vi "Read._Overload.vi"(0 "Index":i32, 1 "Choose_Device":T1(ring), 2 "error in (no error)":errorcluster) -> (3 "Index_Out":i32, 4 "Overload":bool, 5 "Device_type":T1(ring), 6 "error out":errorcluster)   [LabVIEW 2010, in "FEMTO_LUCI-10.lvlib"]
doc: "This function reads the overload of the selected device."
uses:
  <userlib>/FEMTO/FEMTO_LUCI-10.lvlib
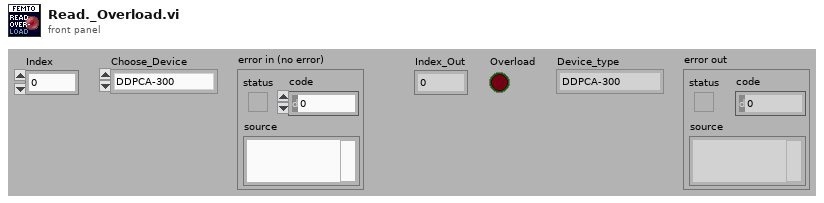
[diagram p1: front panel]
types:
  T1 = enum16{"DDPCA-300", "DLPCA-200", "DHPCA-100", "OE-200", "LIA-MV-150-S", "LIA-MV-150-D", "LIA-MV-200-L", "LIA-MV-200-H", "LIA-MVD-200-L", "LIA-MVD-200-H", "DLPVA-100-BUN-S", "DLPVA-100-BLN-S", "DLPVA-100-B-S", "DLPVA-100-B-D", "DLPVA-100-F-S", "DLPVA-100-F-D", "DHPVA-100", "DHPVA-200", "DUPVA-1-60", "DUPVA-1-70"}
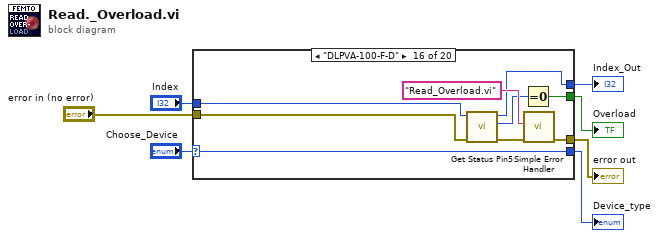
[diagram p0: block diagram]
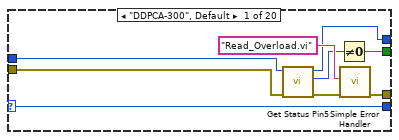
[diagram p2: hidden frame]
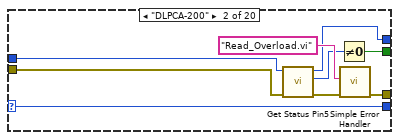
[diagram p3: hidden frame]
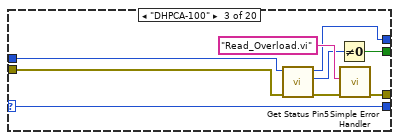
[diagram p4: hidden frame]
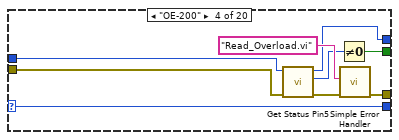
[diagram p5: hidden frame]
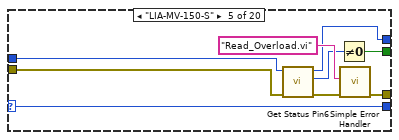
[diagram p6: hidden frame]
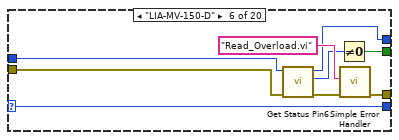
[diagram p7: hidden frame]
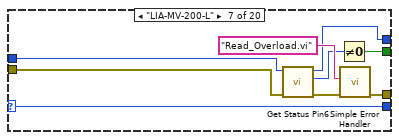
[diagram p8: hidden frame]
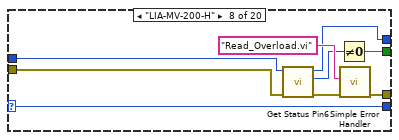
[diagram p9: hidden frame]
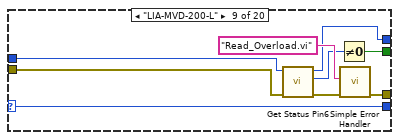
[diagram p10: hidden frame]
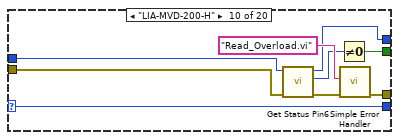
[diagram p11: hidden frame]
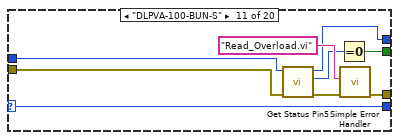
[diagram p12: hidden frame]
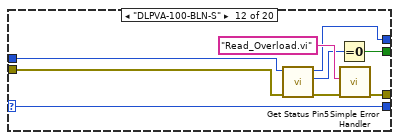
[diagram p13: hidden frame]
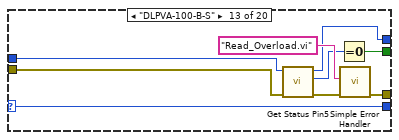
[diagram p14: hidden frame]
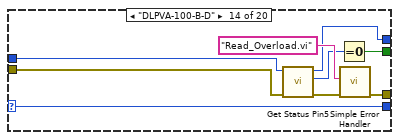
[diagram p15: hidden frame]
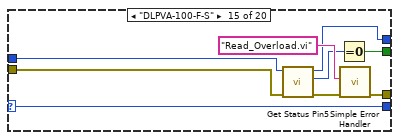
[diagram p16: hidden frame]
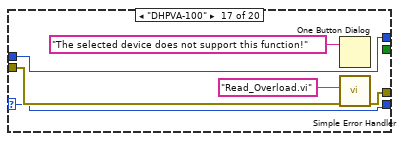
[diagram p17: hidden frame]
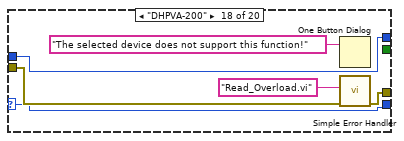
[diagram p18: hidden frame]
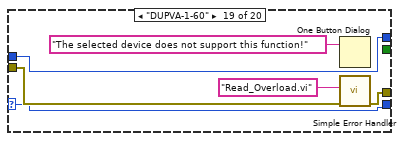
[diagram p19: hidden frame]
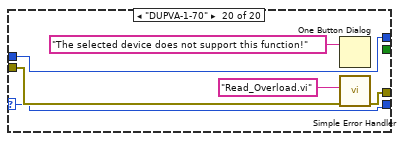
[diagram p20: hidden frame]
diagram:
  n1 = case shown="\"DLPVA-100-F-D\"" "Choose_Device" {
    selector: "Choose_Device" -> [w14 w24 w32 w41 w50 w59 w68 w77 w86 w95 w104 w113 w122 w131 w141 w149 w154 w160 w166 w172]
    tunnel: "error in (no error)" -> [w13 w18 w27 w36 w45 w54 w63 w74 w85 w93 w99 w111 w120 w126 w136 w144 w156 w162 w168 w174]
    tunnel: [w15 w25 w34 w42 w51 w60 w69 w78 w87 w96 w105 w114 w123 w132 w134 w150 w155 w161 w167 w173] -> w3
    tunnel: [w14 w24 w32 w41 w50 w59 w68 w77 w86 w95 w104 w113 w122 w131 w141 w149 w154 w160 w166 w172] -> w4
    tunnel: "Index" -> [w11 w21 w30 w39 w47 w56 w65 w72 w83 w91 w102 w107 w118 w129 w139 w147 w153 w159 w165 w171]
    tunnel: [w10 w20 w29 w38 w46 w55 w64 w71 w82 w90 w101 w108 w117 w128 w138 w146 w153 w159 w165 w171] -> w6
    tunnel: [w8 w19 w28 w37 w48 w57 w66 w75 w80 w89 w100 w109 w116 w127 w137 w145 _ _ _ _] -> w7
    frame "DDPCA-300", Default {
      n2 = call <userlib>:"Get Status Pin5.vi"("error in (no error)"=w13, "index"=w11) -> ("error out"=w12:errorcluster, "status out"=w9:i32, "index_out"=w10:i32)  [unwired: 7 out]
      n3 = Not Equal To 0?(x=w9) -> (x != 0?=w8:bool)
      n4 = call <vilib>:"Simple Error Handler.vi"("error source (\" \")"="Read_Overload.vi" ("error source (\" \")"), "error in (no error)"=w12) -> ("error out"=w15:errorcluster)  [unwired: 1 in, 6 out]
    }
    frame "DLPCA-200" {
      n5 = call <userlib>:"Get Status Pin5.vi"("error in (no error)"=w18, "index"=w21) -> ("error out"=w17:errorcluster, "status out"=w22:i32, "index_out"=w20:i32)  [unwired: 7 out]
      n6 = Not Equal To 0?(x=w22) -> (x != 0?=w19:bool)
      n7 = call <vilib>:"Simple Error Handler.vi"("error source (\" \")"="Read_Overload.vi" ("error source (\" \")"), "error in (no error)"=w17) -> ("error out"=w25:errorcluster)  [unwired: 1 in, 6 out]
    }
    frame "DHPCA-100" {
      n8 = call <userlib>:"Get Status Pin5.vi"("error in (no error)"=w27, "index"=w30) -> ("error out"=w26:errorcluster, "status out"=w31:i32, "index_out"=w29:i32)  [unwired: 7 out]
      n9 = Not Equal To 0?(x=w31) -> (x != 0?=w28:bool)
      n10 = call <vilib>:"Simple Error Handler.vi"("error source (\" \")"="Read_Overload.vi" ("error source (\" \")"), "error in (no error)"=w26) -> ("error out"=w34:errorcluster)  [unwired: 1 in, 6 out]
    }
    frame "OE-200" {
      n11 = call <userlib>:"Get Status Pin5.vi"("error in (no error)"=w36, "index"=w39) -> ("error out"=w35:errorcluster, "status out"=w40:i32, "index_out"=w38:i32)  [unwired: 7 out]
      n12 = Not Equal To 0?(x=w40) -> (x != 0?=w37:bool)
      n13 = call <vilib>:"Simple Error Handler.vi"("error source (\" \")"="Read_Overload.vi" ("error source (\" \")"), "error in (no error)"=w35) -> ("error out"=w42:errorcluster)  [unwired: 1 in, 6 out]
    }
    frame "LIA-MV-150-S" {
      n14 = call <userlib>:"Get Status Pin6.vi"("error in (no error)"=w45, "index"=w47) -> ("error out"=w44:errorcluster, "status out"=w49:i32, "index_out"=w46:i32)  [unwired: 7 out]
      n15 = Not Equal To 0?(x=w49) -> (x != 0?=w48:bool)
      n16 = call <vilib>:"Simple Error Handler.vi"("error source (\" \")"="Read_Overload.vi" ("error source (\" \")"), "error in (no error)"=w44) -> ("error out"=w51:errorcluster)  [unwired: 1 in, 6 out]
    }
    frame "LIA-MV-150-D" {
      n17 = call <userlib>:"Get Status Pin6.vi"("error in (no error)"=w54, "index"=w56) -> ("error out"=w53:errorcluster, "status out"=w58:i32, "index_out"=w55:i32)  [unwired: 7 out]
      n18 = Not Equal To 0?(x=w58) -> (x != 0?=w57:bool)
      n19 = call <vilib>:"Simple Error Handler.vi"("error source (\" \")"="Read_Overload.vi" ("error source (\" \")"), "error in (no error)"=w53) -> ("error out"=w60:errorcluster)  [unwired: 1 in, 6 out]
    }
    frame "LIA-MV-200-L" {
      n20 = call <userlib>:"Get Status Pin6.vi"("error in (no error)"=w63, "index"=w65) -> ("error out"=w62:errorcluster, "status out"=w67:i32, "index_out"=w64:i32)  [unwired: 7 out]
      n21 = Not Equal To 0?(x=w67) -> (x != 0?=w66:bool)
      n22 = call <vilib>:"Simple Error Handler.vi"("error source (\" \")"="Read_Overload.vi" ("error source (\" \")"), "error in (no error)"=w62) -> ("error out"=w69:errorcluster)  [unwired: 1 in, 6 out]
    }
    frame "LIA-MV-200-H" {
      n23 = call <userlib>:"Get Status Pin6.vi"("error in (no error)"=w74, "index"=w72) -> ("error out"=w73:errorcluster, "status out"=w76:i32, "index_out"=w71:i32)  [unwired: 7 out]
      n24 = Not Equal To 0?(x=w76) -> (x != 0?=w75:bool)
      n25 = call <vilib>:"Simple Error Handler.vi"("error source (\" \")"="Read_Overload.vi" ("error source (\" \")"), "error in (no error)"=w73) -> ("error out"=w78:errorcluster)  [unwired: 1 in, 6 out]
    }
    frame "LIA-MVD-200-L" {
      n26 = call <userlib>:"Get Status Pin6.vi"("error in (no error)"=w85, "index"=w83) -> ("error out"=w84:errorcluster, "status out"=w81:i32, "index_out"=w82:i32)  [unwired: 7 out]
      n27 = Not Equal To 0?(x=w81) -> (x != 0?=w80:bool)
      n28 = call <vilib>:"Simple Error Handler.vi"("error source (\" \")"="Read_Overload.vi" ("error source (\" \")"), "error in (no error)"=w84) -> ("error out"=w87:errorcluster)  [unwired: 1 in, 6 out]
    }
    frame "LIA-MVD-200-H" {
      n29 = call <userlib>:"Get Status Pin6.vi"("error in (no error)"=w93, "index"=w91) -> ("error out"=w92:errorcluster, "status out"=w94:i32, "index_out"=w90:i32)  [unwired: 7 out]
      n30 = Not Equal To 0?(x=w94) -> (x != 0?=w89:bool)
      n31 = call <vilib>:"Simple Error Handler.vi"("error source (\" \")"="Read_Overload.vi" ("error source (\" \")"), "error in (no error)"=w92) -> ("error out"=w96:errorcluster)  [unwired: 2 in, 5 out]
    }
    frame "DLPVA-100-BUN-S" {
      n32 = call <userlib>:"Get Status Pin5.vi"("error in (no error)"=w99, "index"=w102) -> ("error out"=w98:errorcluster, "status out"=w103:i32, "index_out"=w101:i32)  [unwired: 7 out]
      n33 = Equal To 0?(x=w103) -> (x = 0?=w100:bool)
      n34 = call <vilib>:"Simple Error Handler.vi"("error source (\" \")"="Read_Overload.vi" ("error source (\" \")"), "error in (no error)"=w98) -> ("error out"=w105:errorcluster)  [unwired: 1 in, 6 out]
    }
    frame "DLPVA-100-BLN-S" {
      n35 = call <userlib>:"Get Status Pin5.vi"("error in (no error)"=w111, "index"=w107) -> ("error out"=w110:errorcluster, "status out"=w112:i32, "index_out"=w108:i32)  [unwired: 7 out]
      n36 = Equal To 0?(x=w112) -> (x = 0?=w109:bool)
      n37 = call <vilib>:"Simple Error Handler.vi"("error source (\" \")"="Read_Overload.vi" ("error source (\" \")"), "error in (no error)"=w110) -> ("error out"=w114:errorcluster)  [unwired: 1 in, 6 out]
    }
    frame "DLPVA-100-B-S" {
      n38 = call <userlib>:"Get Status Pin5.vi"("error in (no error)"=w120, "index"=w118) -> ("error out"=w119:errorcluster, "status out"=w121:i32, "index_out"=w117:i32)  [unwired: 7 out]
      n39 = Equal To 0?(x=w121) -> (x = 0?=w116:bool)
      n40 = call <vilib>:"Simple Error Handler.vi"("error source (\" \")"="Read_Overload.vi" ("error source (\" \")"), "error in (no error)"=w119) -> ("error out"=w123:errorcluster)  [unwired: 1 in, 6 out]
    }
    frame "DLPVA-100-B-D" {
      n41 = call <userlib>:"Get Status Pin5.vi"("error in (no error)"=w126, "index"=w129) -> ("error out"=w125:errorcluster, "status out"=w130:i32, "index_out"=w128:i32)  [unwired: 7 out]
      n42 = Equal To 0?(x=w130) -> (x = 0?=w127:bool)
      n43 = call <vilib>:"Simple Error Handler.vi"("error source (\" \")"="Read_Overload.vi" ("error source (\" \")"), "error in (no error)"=w125) -> ("error out"=w132:errorcluster)  [unwired: 1 in, 6 out]
    }
    frame "DLPVA-100-F-S" {
      n44 = call <userlib>:"Get Status Pin5.vi"("error in (no error)"=w136, "index"=w139) -> ("error out"=w135:errorcluster, "status out"=w140:i32, "index_out"=w138:i32)  [unwired: 7 out]
      n45 = Equal To 0?(x=w140) -> (x = 0?=w137:bool)
      n46 = call <vilib>:"Simple Error Handler.vi"("error source (\" \")"="Read_Overload.vi" ("error source (\" \")"), "error in (no error)"=w135) -> ("error out"=w134:errorcluster)  [unwired: 1 in, 6 out]
    }
    frame "DLPVA-100-F-D" {
      n47 = call <userlib>:"Get Status Pin5.vi"("error in (no error)"=w144, "index"=w147) -> ("error out"=w143:errorcluster, "status out"=w148:i32, "index_out"=w146:i32)  [unwired: 7 out]
      n48 = Equal To 0?(x=w148) -> (x = 0?=w145:bool)
      n49 = call <vilib>:"Simple Error Handler.vi"("error source (\" \")"="Read_Overload.vi" ("error source (\" \")"), "error in (no error)"=w143) -> ("error out"=w150:errorcluster)  [unwired: 1 in, 6 out]
    }
    frame "DHPVA-100" {
      n50 = One Button Dialog(message="The selected device does not support this function!") -> ()  [unwired: 2 out]
      n51 = call <vilib>:"Simple Error Handler.vi"("error source (\" \")"="Read_Overload.vi" ("error source (\" \")"), "error in (no error)"=w156) -> ("error out"=w155:errorcluster)  [unwired: 1 in, 6 out]
    }
    frame "DHPVA-200" {
      n52 = One Button Dialog(message="The selected device does not support this function!") -> ()  [unwired: 2 out]
      n53 = call <vilib>:"Simple Error Handler.vi"("error source (\" \")"="Read_Overload.vi" ("error source (\" \")"), "error in (no error)"=w162) -> ("error out"=w161:errorcluster)  [unwired: 1 in, 6 out]
    }
    frame "DUPVA-1-60" {
      n54 = One Button Dialog(message="The selected device does not support this function!") -> ()  [unwired: 2 out]
      n55 = call <vilib>:"Simple Error Handler.vi"("error source (\" \")"="Read_Overload.vi" ("error source (\" \")"), "error in (no error)"=w168) -> ("error out"=w167:errorcluster)  [unwired: 1 in, 6 out]
    }
    frame "DUPVA-1-70" {
      n56 = One Button Dialog(message="The selected device does not support this function!") -> ()  [unwired: 2 out]
      n57 = call <vilib>:"Simple Error Handler.vi"("error source (\" \")"="Read_Overload.vi" ("error source (\" \")"), "error in (no error)"=w174) -> ("error out"=w173:errorcluster)  [unwired: 1 in, 6 out]
    }
  }
  "error out" <- w3
  "Device_type" <- w4
  "Index_Out" <- w6
  "Overload" <- w7
